vi "ProjectVersionCheck_Global_Init.vi"(11 "Object":T1) -> ()   [LabVIEW 2015]
uses:
  <resource>/Framework/Providers/API/ItemRef.ctl
  <resource>/Framework/Providers/API/mxLvMenuItem.ctl
  LV Project Version Check.lvlib
panel:
  out "error out":errorcluster
  in  "error in":errorcluster
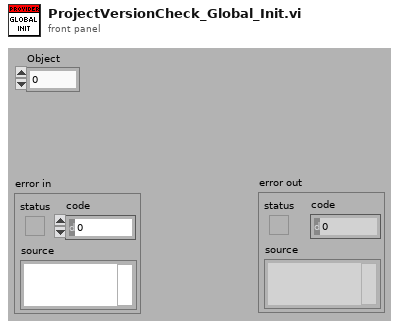
[diagram p1: front panel]
types:
  T1 = typedef "ItemRef.ctl" = u64
  T2 = typedef "mxLvMenuItem.ctl" = cluster{"Menu Name":string, "Description":string, "Icon File Name":path, "Menu Tag":string, "Enabled":bool, "Checked":bool, "Separator":bool, "Batchable":bool, "Weight":i32, "Batch Mode (Ignored if Not Batchable)":enum32{"Show If All Items Support Command", "Show If Any Items Support Command"}, "Menu Location":enum32{"<None>", "Project", "Project / Build Specifications", "Tools", "Tools / Source Control", "Tools / Real-Time Module", "Help"}, "Exclude From Getting Started Window Menu":bool}
  T3 = enum32{"<None>", "Project", "Project / Build Specifications", "Tools", "Tools / Source Control", "Tools / Real-Time Module", "Help"}
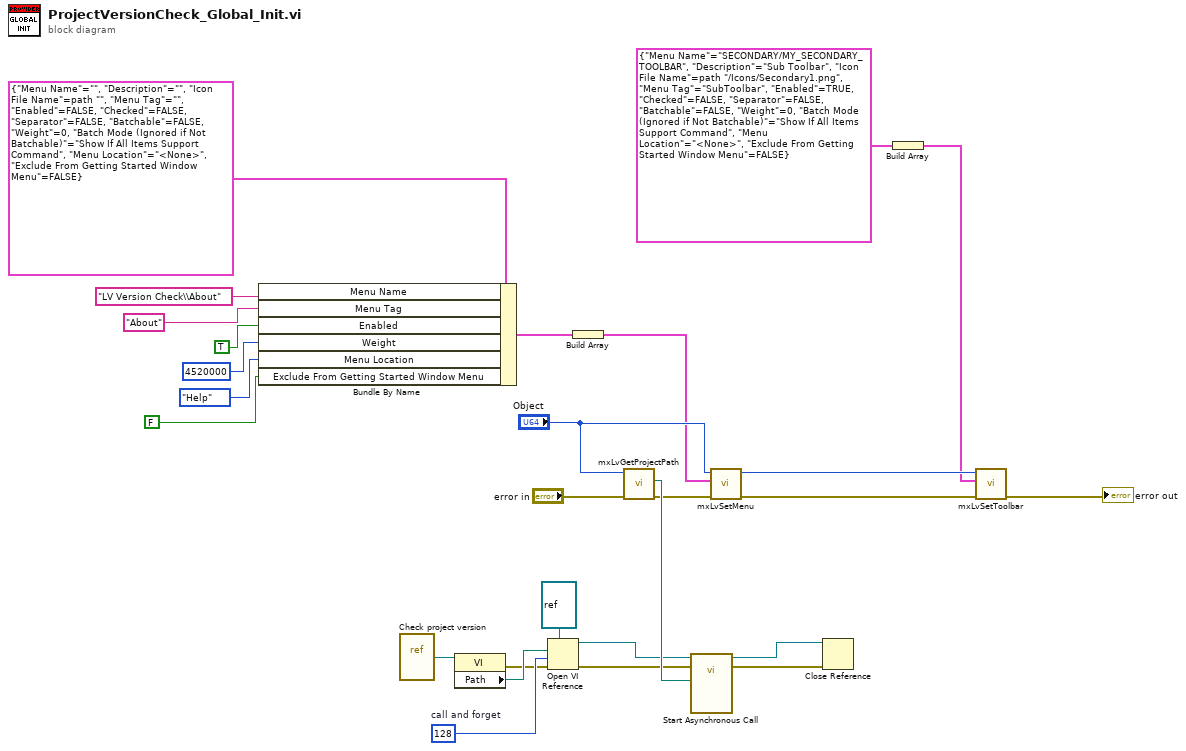
[diagram p0: block diagram]
diagram:
  w9 = 128  # call and forget
  n1 = Bundle By Name(cluster=T2 {"Menu Name"="", "Description"="", "Icon File Name"=path "", "Menu Tag"="", "Enabled"=FALSE, "Checked"=FALSE, "Separator"=FALSE, "Batchable"=FALSE, "Weight"=0, "Batch Mode (Ignored if Not Batchable)"=enum."Show If All Items Support Command", "Menu Location"=enum."<None>", "Exclude From Getting Started Window Menu"=FALSE} ("Menu Item"), "Menu Name"="LV Version Check\\About" ("element"), "Menu Tag"="About" ("menu tag"), "Enabled"=TRUE ("Checked"), "Weight"=4520000 ("menu weight"), "Menu Location"=T3."Help", "Exclude From Getting Started Window Menu"=FALSE) -> (w11:T2)
  n2 = vi-ref "Check project version.vi"() -> (w3:refnum<vi>)
  n3 = property class="VI"(reference=w3) -> (error out=w1:errorcluster, "Path"=w2:path)  [unwired: 1 in, 1 out]
  n4 = Open VI Reference(type specifier VI Refnum (for type only)=refnum<vi> refnum, vi path=w2, options=w9, error in (no error)=w1) -> (vi reference=w7:refnum<vi>, error out=w6:errorcluster)  [unwired: 2 in]
  n5 = Build Array(w11) -> (w10:T2[])
  n6 = call <resource>:"mxLvGetProjectPath.vi"("error in"="error in", "Item"="Object") -> ("error out"=w23:errorcluster, "Project Path"=w26:path)  [unwired: 7 in, 1 out]
  n7 = call-by-ref "Start Asynchronous Call"(reference=w7, error in=w6, "path to XML document"=w26) -> (reference out=w4:refnum<vi>, error out=w5:errorcluster)  [unwired: 10 in, 1 out]
  n8 = call <resource>:"mxLvSetMenu.vi"("error in"=w23, "Menu Items"=w10, "Item"="Object") -> ("error out"=w24:errorcluster, "Item"=w25:T1)  [unwired: 7 out]
  n9 = Close Reference(reference=w4, error in (no error)=w5) -> ()  [unwired: 1 out]
  n10 = Build Array(T2 {"Menu Name"="SECONDARY/MY_SECONDARY_TOOLBAR", "Description"="Sub Toolbar", "Icon File Name"=path "../Icons/Secondary1.png", "Menu Tag"="SubToolbar", "Enabled"=TRUE, "Checked"=FALSE, "Separator"=FALSE, "Batchable"=FALSE, "Weight"=0, "Batch Mode (Ignored if Not Batchable)"=enum."Show If All Items Support Command", "Menu Location"=enum."<None>", "Exclude From Getting Started Window Menu"=FALSE} ("Menu Item")) -> (w19:T2[])
  n11 = call <resource>:"mxLvSetToolbar.vi"("error in"=w24, "Toolbar Items"=w19, "Item"=w25) -> ("error out"=→"error out":errorcluster)  [unwired: 7 in, 1 out]
